vi "Write Image Name Prefix.vi"(8 "error in (no error)":errorcluster, 10 "Image Name Prefix":string, 11 "AF IMAQ Display in":refnum<class "HIJ Vision Display.lvclass">) -> (0 "error out":errorcluster, 3 "AF IMAQ Display out":refnum<class "HIJ Vision Display.lvclass">)   [LabVIEW 2014, in "HIJ Vision Display.lvlib" / "HIJ Vision Display.lvclass"]
uses:
  HIJ Vision Display.lvclass
  HIJ Vision Display.lvclass/HIJ Vision Display.ctl
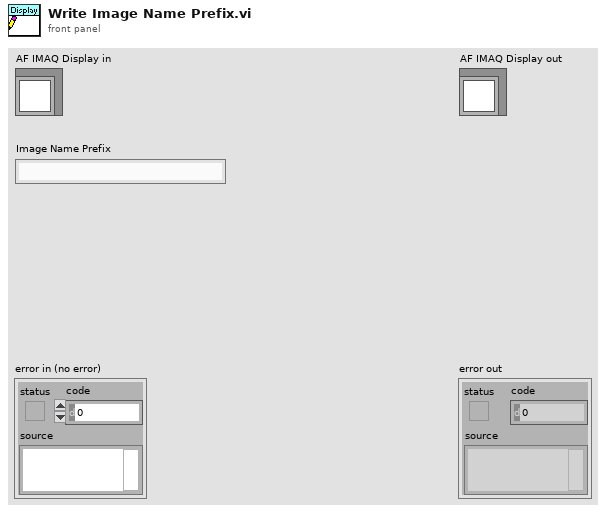
[diagram p1: front panel]
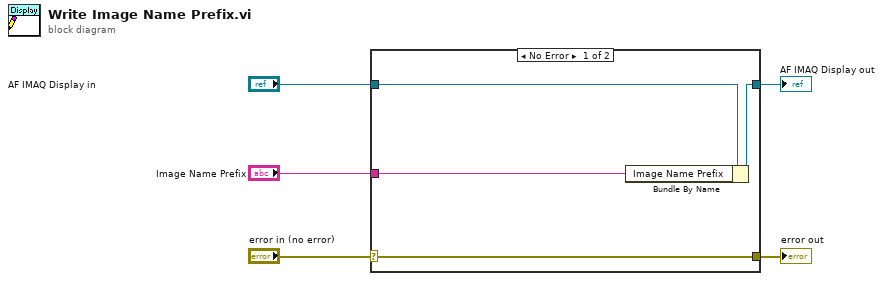
[diagram p0: block diagram]
diagram:
  n1 = case shown="No Error" "error in (no error)" {
    selector: "error in (no error)" -> [w9 w10]
    tunnel: [w9 w10] -> w4
    tunnel: [w7 w11] -> w2
    tunnel: "AF IMAQ Display in" -> [w8 w11]
    tunnel: "Image Name Prefix" -> [w6 _]
    frame No Error {
      n2 = Bundle By Name(cluster=w8, "Image Name Prefix"=w6) -> (w7:refnum<class "HIJ Vision Display.lvclass">)
    }
    frame Error {
    }
  }
  "error out" <- w4
  "AF IMAQ Display out" <- w2
